vi "Update Measurement Results.vi"(0 "measurement results in":T3, 1 "measurement configuration":T1={"Mode of operation"=enum."Perform measurement", "DUT setup time"=1.0, "Source delay"=0.005, "Aperture time"=0.005, "Nominal output voltage"=3.3, "Source pin name"="", "Source sense"=1009, "Source current limit"=25.0, "Source maximum power"=300.0, "Source start voltage"=6.0, "Source stop voltage"=20.0, "Source voltage sweep points"=4, "Use Source voltage array"=FALSE, "Source voltage array"=[], "Load pin name"="", "Load sense"=1009, "Load voltage limit range"=6.0, "Load sweep type"="Logarithmic", "Load start current"=0.1, "Load stop current"=24.0, "Load current sweep points/points per decade"=10, "Use Load current array"=FALSE, "Load current array"=[], "Pin Names for Scope"=[], "vertical range"=[], "vertical offset"=[], "probe attenuation"=[], "vertical coupling"=[], "channel enabled"=[], "input impedance"=[], "max input frequency"=[], "min sample rate"=[], "reference position"=[], "min record length"=[], "enforce realtime"=[]} {"input impedance" items=["1 mega ohm"=0, "50 ohms"=2]; "vertical coupling" items=["AC", "DC", "Ground"]; "Load sense" items=["Local"=1008, "Remote"=1009]; "Source sense" items=["Local"=1008, "Remote"=1009]}, 2 "waveform pins":string[](array[string]), 3 "waveform sites":i32[](array[numeric]), 4 "Scope waveforms":waveform(dbl)[](array[waveform]), 5 "error in (no error)":errorcluster, 6 "Load currents":dbl[](array[numeric]), 8 "Load voltages":dbl[](array[numeric]), 10 "Source currents":dbl[](array[numeric]), 12 "Source voltages":dbl[](array[numeric])) -> (14 "measurement results out":T3, 19 "error out":errorcluster)   [LabVIEW 2021, in "Efficiency And Load Regulation with Pin Map.lvlib"]
uses:
  Efficiency And Load Regulation with Pin Map.lvlib
  Measurement Results.ctl
  Measurement Configuration.ctl
  <instrlib>/niScope/Controls/niScope vertical coupling.ctl
  common/builds/PMIC Common.lvlibp
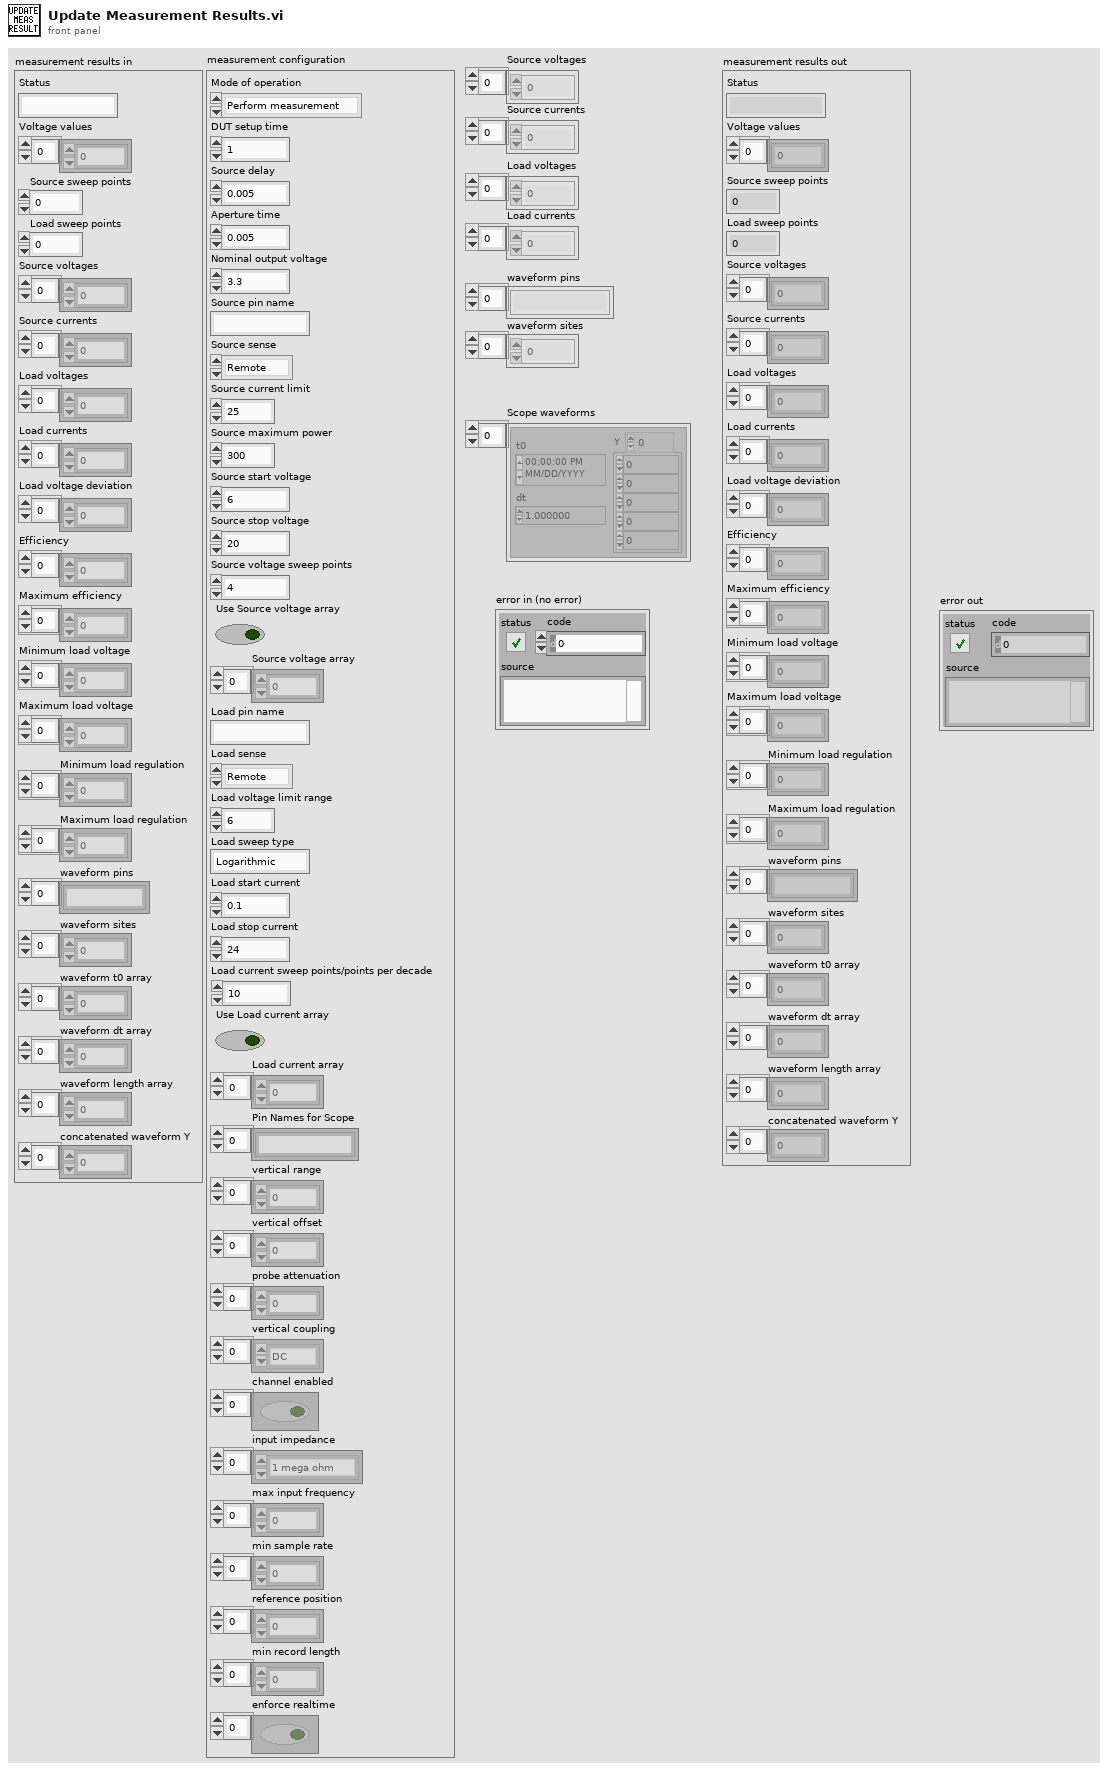
[diagram p1: front panel]
types:
  T1 = typedef "Efficiency And Load Regulation with Pin Map.lvlib/Measurement Configuration.ctl" = cluster{"Mode of operation":enum32{"Power on the DUT", "Perform measurement", "Power off the DUT"}, "DUT setup time":dbl, "Source delay":dbl, "Aperture time":dbl, "Nominal output voltage":dbl, "Source pin name":string, "Source sense":i32, "Source current limit":dbl, "Source maximum power":dbl, "Source start voltage":dbl, "Source stop voltage":dbl, "Source voltage sweep points":i32, "Use Source voltage array":bool, "Source voltage array":dbl[], "Load pin name":string, "Load sense":i32, "Load voltage limit range":dbl, "Load sweep type":string, "Load start current":dbl, "Load stop current":dbl, "Load current sweep points/points per decade":i32, "Use Load current array":bool, "Load current array":dbl[], "Pin Names for Scope":string[], "vertical range":dbl[], "vertical offset":dbl[], "probe attenuation":dbl[], "vertical coupling":T2[], "channel enabled":bool[], "input impedance":u32[], "max input frequency":dbl[], "min sample rate":dbl[], "reference position":dbl[], "min record length":i32[], "enforce realtime":bool[]}
  T2 = typedef "niScope vertical coupling.ctl" = i32
  T3 = typedef "Efficiency And Load Regulation with Pin Map.lvlib/Measurement Results.ctl" = cluster{"Status":string, "Voltage values":dbl[], "Source sweep points":i32, "Load sweep points":i32, "Source voltages":dbl[], "Source currents":dbl[], "Load voltages":dbl[], "Load currents":dbl[], "Load voltage deviation":dbl[], "Efficiency":dbl[], "Maximum efficiency":dbl[], "Minimum load voltage":dbl[], "Maximum load voltage":dbl[], "Minimum load regulation":dbl[], "Maximum load regulation":dbl[], "waveform pins":string[], "waveform sites":i32[], "waveform t0 array":dbl[], "waveform dt array":dbl[], "waveform length array":i32[], "concatenated waveform Y":dbl[]}
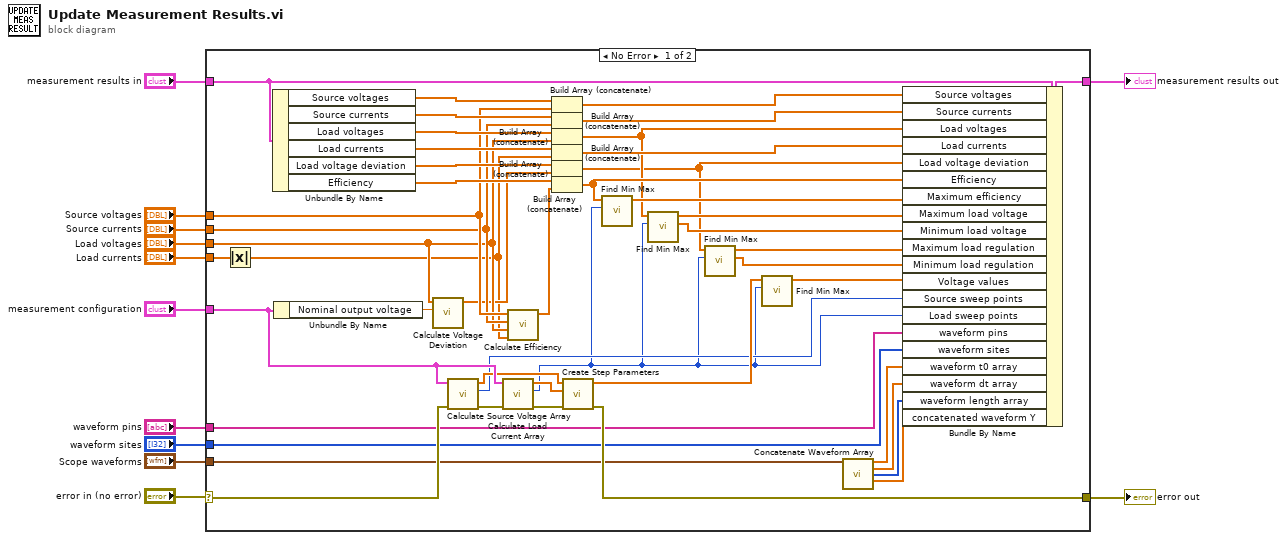
[diagram p0: block diagram]
diagram:
  n1 = case shown="No Error" "error in (no error)" {
    selector: "error in (no error)" -> [w23 w59]
    tunnel: "measurement results in" -> [w57 w58]
    tunnel: "Source voltages" -> [w45 _]
    tunnel: "Source currents" -> [w44 _]
    tunnel: "Load voltages" -> [w43 _]
    tunnel: "Load currents" -> [w41 _]
    tunnel: [w40 w58] -> w7
    tunnel: "measurement configuration" -> [w30 _]
    tunnel: "Scope waveforms" -> [w19 _]
    tunnel: [w24 w59] -> w4
    tunnel: "waveform pins" -> [w14 _]
    tunnel: "waveform sites" -> [w13 _]
    frame No Error {
      n2 = Absolute Value(x=w41) -> (abs(x)=w22:dbl[])
      n3 = Unbundle By Name(w57) -> ("Source voltages"=w56:dbl[], "Source currents"=w55:dbl[], "Load voltages"=w54:dbl[], "Load currents"=w53:dbl[], "Load voltage deviation"=w48:dbl[], "Efficiency"=w47:dbl[])
      n4 = Unbundle By Name(w30) -> ("Nominal output voltage"=w49:dbl)
      n5 = call "Calculate Voltage Deviation.vi"("Nominal output voltage"=w49, "Voltage measurements"=w43) -> ("Load voltage deviation"=w42:dbl[])  [unwired: 9 in]
      n6 = call "Calculate Source Voltage Array.vi"("error in"=w23, "measurement configuration"=w30) -> ("error out"=w31:errorcluster, "Source voltage array size"=w21:i32, "Source voltage array"=w27:dbl[])  [unwired: 7 in]
      n7 = call "Calculate Load Current Array.vi"("error in"=w31, "measurement configuration"=w30) -> ("error out"=w29:errorcluster, "Load current array size"=w20:i32, "Load current array"=w28:dbl[])  [unwired: 7 in]
      n8 = call "Calculate Efficiency.vi"("load current measurements"=w22, "load voltage measurements"=w43, "source current measurements"=w44, "source voltage measurements"=w45) -> ("Efficiency(%)"=w46:dbl[])  [unwired: 7 in]
      n9 = Build Array (concatenate)(w56, w45) -> (w52:dbl[])
      n10 = Build Array (concatenate)(w55, w44) -> (w51:dbl[])
      n11 = Build Array (concatenate)(w54, w43) -> (w35:dbl[])
      n12 = Build Array (concatenate)(w53, w22) -> (w50:dbl[])
      n13 = Build Array (concatenate)(w48, w42) -> (w32:dbl[])
      n14 = Build Array (concatenate)(w47, w46) -> (w38:dbl[])
      n15 = call "Create Step Parameters.vi"("error in (no error)"=w29, "Load current array"=w28, "Source voltage array"=w27) -> ("error out"=w24:errorcluster, "Source voltage values"=w25:dbl[])  [unwired: 5 in, 2 out]
      n16 = call "Find Min Max.vi"("chunk size"=w20, "Input Array"=w38) -> ("Max array"=w39:dbl[])  [unwired: 8 in, 1 out]
      n17 = call "Find Min Max.vi"("chunk size"=w20, "Input Array"=w35) -> ("Min array"=w36:dbl[], "Max array"=w37:dbl[])  [unwired: 8 in]
      n18 = call "Find Min Max.vi"("chunk size"=w20, "Input Array"=w32) -> ("Min array"=w33:dbl[], "Max array"=w34:dbl[])  [unwired: 8 in]
      n19 = call "Find Min Max.vi"("chunk size"=w20, "Input Array"=w25) -> ("Max array"=w26:dbl[])  [unwired: 8 in, 1 out]
      n20 = call "Concatenate Waveform Array.vi"("waveform array"=w19) -> ("waveform t0 array"=w18:dbl[], "waveform dt array"=w17:dbl[], "waveform length array"=w16:i32[], "concatenated waveform Y"=w15:dbl[])  [unwired: 11 in]
      n21 = Bundle By Name(cluster=w57, "Source voltages"=w52, "Source currents"=w51, "Load voltages"=w35, "Load currents"=w50, "Load voltage deviation"=w32, "Efficiency"=w38, "Maximum efficiency"=w39, "Maximum load voltage"=w37, "Minimum load voltage"=w36, "Maximum load regulation"=w34, "Minimum load regulation"=w33, "Voltage values"=w26, "Source sweep points"=w21, "Load sweep points"=w20, "waveform pins"=w14, "waveform sites"=w13, "waveform t0 array"=w18, "waveform dt array"=w17, "waveform length array"=w16, "concatenated waveform Y"=w15) -> (w40:T3)
    }
    frame Error {
    }
  }
  "measurement results out" <- w7
  "error out" <- w4
